vi "selectSummaryData.vi"(10 "End Date":string="2014/9/24", 11 "From Date":string="2014/9/20") -> (3 "Summary":string[][](array[string]))   [LabVIEW 2012]
uses:
  <vilib>/addons/database/Auxilliary.llb/DB Tools Cursor Type.ctl
  Global1.vi
  <vilib>/addons/database/Connection.llb/DB Tools Open Connec (Path).vi
  <vilib>/addons/database/Connection.llb/Conn Execute.vi
  <vilib>/addons/database/Recordset.llb/Rec Fetch Recordset Data (R).vi
  <vilib>/addons/database/Recordset.llb/Rec Destroy - Connection.vi
  <vilib>/addons/database/_DB Variant To Data/Database Variant To Data.xnode
  <vilib>/addons/database/NI_Database_API.lvlib
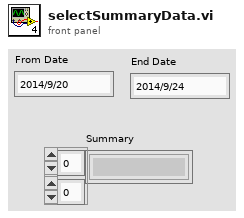
[diagram p1: front panel]
types:
  T1 = typedef "NI_Database_API.lvlib/DB Tools Cursor Type.ctl" = enum16{"forward-only", "keyset", "dynamic", "static"}
  T2 = typedef "NI_Database_API.lvlib/Conn ObjectReference.ctl" = refnum<k1>
  T3 = typedef "NI_Database_API.lvlib/Rec ObjectReference.ctl" = refnum<k1>
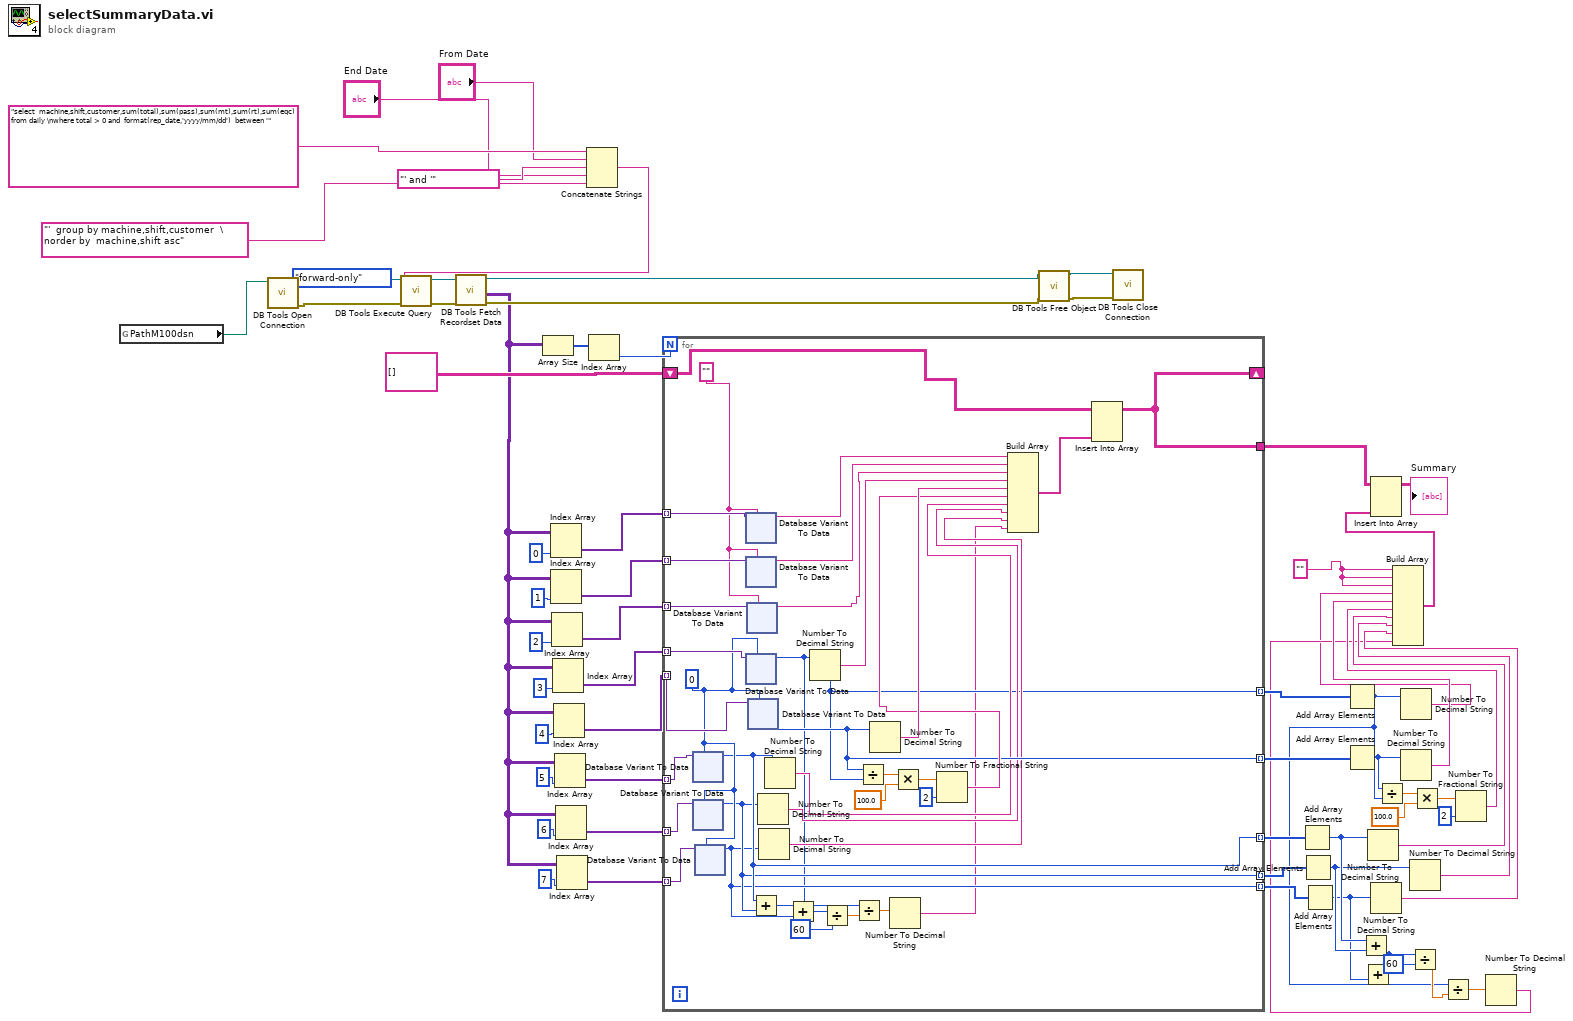
[diagram p0: block diagram]
diagram:
  w48 = "" ("element")
  n1 = global read "Global1.vi" "PathM100dsn"() -> (w1:path)
  n2 = call-poly <vilib>:"DB Tools Open Connection.vi"("connection information"=w1) -> ("error out"=w36:errorcluster, "connection reference"=w37:T2)  [unwired: 7 in]
  n3 = Concatenate Strings("select  machine,shift,customer,sum(total),sum(pass),sum(mt),sum(rt),sum(eqc) from daily \nwhere total > 0 and  format(rep_date,'yyyy/mm/dd')  between '" ("string"), "From Date", "' and '" ("string"), "End Date", "'  group by machine,shift,customer  \norder by  machine,shift asc" ("string")) -> (w33:string)
  n4 = call-poly <vilib>:"DB Tools Execute Query.vi"("error in (no error)"=w36, "cursor type"=DB_Tools_Cursor_Type."forward-only", "SQL query"=w33, "connection reference"=w37) -> ("error out"=w39:errorcluster, "recordset reference"=w38:T3)  [unwired: 4 in]
  n5 = call-poly <vilib>:"DB Tools Fetch Recordset Data.vi"("error in (no error)"=w39, "recordset reference"=w38) -> ("error out"=w35:errorcluster, "recordset data"=w24:variant[][], "recordset reference out"=w34:T3)  [unwired: 3 in]
  n6 = Array Size(array=w24) -> (size(s)=w65:i32[])
  n7 = Index Array(array=w24, index (col)=0) -> (element=w58:variant[])  [unwired: 1 in]
  n8 = Index Array(array=w24, index (col)=1) -> (element=w57:variant[])  [unwired: 1 in]
  n9 = Index Array(array=w24, index (col)=2) -> (element=w53:variant[])  [unwired: 1 in]
  n10 = Index Array(array=w24, index (col)=3) -> (element=w56:variant[])  [unwired: 1 in]
  n11 = Index Array(array=w24, index (col)=4) -> (element=w55:variant[])  [unwired: 1 in]
  n12 = Index Array(array=w24, index (col)=5) -> (element=w23:variant[])  [unwired: 1 in]
  n13 = Index Array(array=w24, index (col)=6) -> (element=w22:variant[])  [unwired: 1 in]
  n14 = Index Array(array=w24, index (col)=7) -> (element=w21:variant[])  [unwired: 1 in]
  n15 = Index Array(array=w65) -> (element=w64:i32)  [unwired: 1 in]
  n16 = for {
    N: w64 -> [_]
    tunnel: w55 -> [w102] mode=indexing
    shift-right: [w83] -> _
    shift-left: string[][] [] -> [w87]
    tunnel: w58 -> [w101] mode=indexing
    tunnel: w57 -> [w100] mode=indexing
    tunnel: w56 -> [w99] mode=indexing
    tunnel: w53 -> [w96] mode=indexing
    tunnel: [w68] -> w11 mode=indexing
    tunnel: [w89] -> w51 mode=indexing
    tunnel: [w83] -> w31
    tunnel: w23 -> [w82] mode=indexing
    tunnel: w22 -> [w81] mode=indexing
    tunnel: w21 -> [w80] mode=indexing
    tunnel: [w72] -> w18 mode=indexing
    tunnel: [w74] -> w19 mode=indexing
    tunnel: [w75] -> w20 mode=indexing
    w79 = 0
    w95 = ""
    n17 = xnode "Database Variant To Data"("database variant"=w82, "type"=w79) -> ("data"=w75:i32)  [unwired: 1 in, 1 out]
    n18 = xnode "Database Variant To Data"("database variant"=w81, "type"=w79) -> ("data"=w74:i32)  [unwired: 1 in, 1 out]
    n19 = xnode "Database Variant To Data"("database variant"=w80, "type"=w79) -> ("data"=w72:i32)  [unwired: 1 in, 1 out]
    n20 = xnode "Database Variant To Data"("database variant"=w101, "type"=w95) -> ("data"=w86:string)  [unwired: 1 in, 1 out]
    n21 = xnode "Database Variant To Data"("database variant"=w100, "type"=w95) -> ("data"=w85:string)  [unwired: 1 in, 1 out]
    n22 = xnode "Database Variant To Data"("database variant"=w99, "type"=w79) -> ("data"=w68:i32)  [unwired: 1 in, 1 out]
    n23 = xnode "Database Variant To Data"("database variant"=w96, "type"=w95) -> ("data"=w84:string)  [unwired: 1 in, 1 out]
    n24 = xnode "Database Variant To Data"("database variant"=w102, "type"=w79) -> ("data"=w89:i32)  [unwired: 1 in, 1 out]
    n25 = Add(x=w75, y=w74) -> (x+y=w73:i32)
    n26 = Number To Decimal String(number=w74) -> (decimal integer string=w77:string)  [unwired: 1 in]
    n27 = Number To Decimal String(number=w72) -> (decimal integer string=w76:string)  [unwired: 1 in]
    n28 = Number To Decimal String(number=w75) -> (decimal integer string=w78:string)  [unwired: 1 in]
    n29 = Add(x=w73, y=w72) -> (x+y=w71:i32)
    n30 = Number To Decimal String(number=w68) -> (decimal integer string=w93:string)  [unwired: 1 in]
    n31 = Divide(x=w71, y=60) -> (x/y=w69:dbl)
    n32 = Divide(x=w68, y=w69) -> (x/y=w67:dbl)
    n33 = Divide(x=w89, y=w68) -> (x/y=w97:dbl)
    n34 = Number To Decimal String(number=w89) -> (decimal integer string=w94:string)  [unwired: 1 in]
    n35 = Number To Decimal String(number=w67) -> (decimal integer string=w66:string)  [unwired: 1 in]
    n36 = Multiply(x=w97, y=100.0) -> (x*y=w92:dbl)
    n37 = Number To Fractional String(number=w92, precision (6)=i16 2) -> (F-format string=w91:string)  [unwired: 2 in]
    n38 = Build Array(w86, w85, w84, w93, w94, w91, w78, w77, w76, w66) -> (w88:string[])
    n39 = Insert Into Array(array=w87, new element=w88) -> (w83:string[][])  [unwired: 2 in]
  }
  n40 = call-poly <vilib>:"DB Tools Free Object.vi"("error in (no error)"=w35, "recordset reference"=w34) -> ("error out"=w40:errorcluster, "connection reference"=w41:T2)  [unwired: 8 in]
  n41 = call <vilib>:"DB Tools Close Connection.vi"("error in (no error)"=w40, "connection reference"=w41) -> ()  [unwired: 5 in, 1 out]
  n42 = Add Array Elements(numeric array=w20) -> (sum=w14:i32)
  n43 = Add Array Elements(numeric array=w19) -> (sum=w13:i32)
  n44 = Add Array Elements(numeric array=w18) -> (sum=w12:i32)
  n45 = Add Array Elements(numeric array=w11) -> (sum=w5:i32)
  n46 = Add Array Elements(numeric array=w51) -> (sum=w43:i32)
  n47 = Add(x=w14, y=w13) -> (x+y=w10:i32)
  n48 = Add(x=w10, y=w12) -> ()  [unwired: 1 out]
  n49 = Number To Decimal String(number=w14) -> (decimal integer string=w17:string)  [unwired: 1 in]
  n50 = Number To Decimal String(number=w12) -> (decimal integer string=w15:string)  [unwired: 1 in]
  n51 = Divide(x=w43, y=w5) -> (x/y=w46:dbl)
  n52 = Number To Decimal String(number=w5) -> (decimal integer string=w3:string)  [unwired: 1 in]
  n53 = Number To Decimal String(number=w43) -> (decimal integer string=w50:string)  [unwired: 1 in]
  n54 = Number To Decimal String(number=w13) -> (decimal integer string=w16:string)  [unwired: 1 in]
  n55 = Divide(x=w10, y=60) -> (x/y=w8:dbl)
  n56 = Multiply(x=w46, y=100.0) -> (x*y=w45:dbl)
  n57 = Divide(x=w5, y=w8) -> (x/y=w7:dbl)
  n58 = Number To Fractional String(number=w45, precision (6)=i16 2) -> (F-format string=w42:string)  [unwired: 2 in]
  n59 = Number To Decimal String(number=w7) -> (decimal integer string=w6:string)  [unwired: 1 in]
  n60 = Build Array(w48, w48, w48, w3, w50, w42, w17, w16, w15, w6) -> (w49:string[])
  n61 = Insert Into Array(array=w31, new element=w49) -> (→"Summary":string[][])  [unwired: 2 in]
